vi "lab_3_partie_4.vi"() -> ()   [LabVIEW 2020]
uses:
  <instrlib>/Agilent 34401/Public/Data/Read (Single Point).vi
  <instrlib>/Agilent E363X Series/Agilent E363X Series.lvlib
  <instrlib>/Agilent 34401/Agilent 34401.lvlib
panel:
  out "XY Graph":cluster{"Y":dbl[], "Y":dbl[]}[](graph) caption="Graphe XY"
  in  "Tension maximale":dbl(slide) scale=0.0..6.0
  out "Courant":dbl
  in  "Incrément \ntension":sgl step=0.05
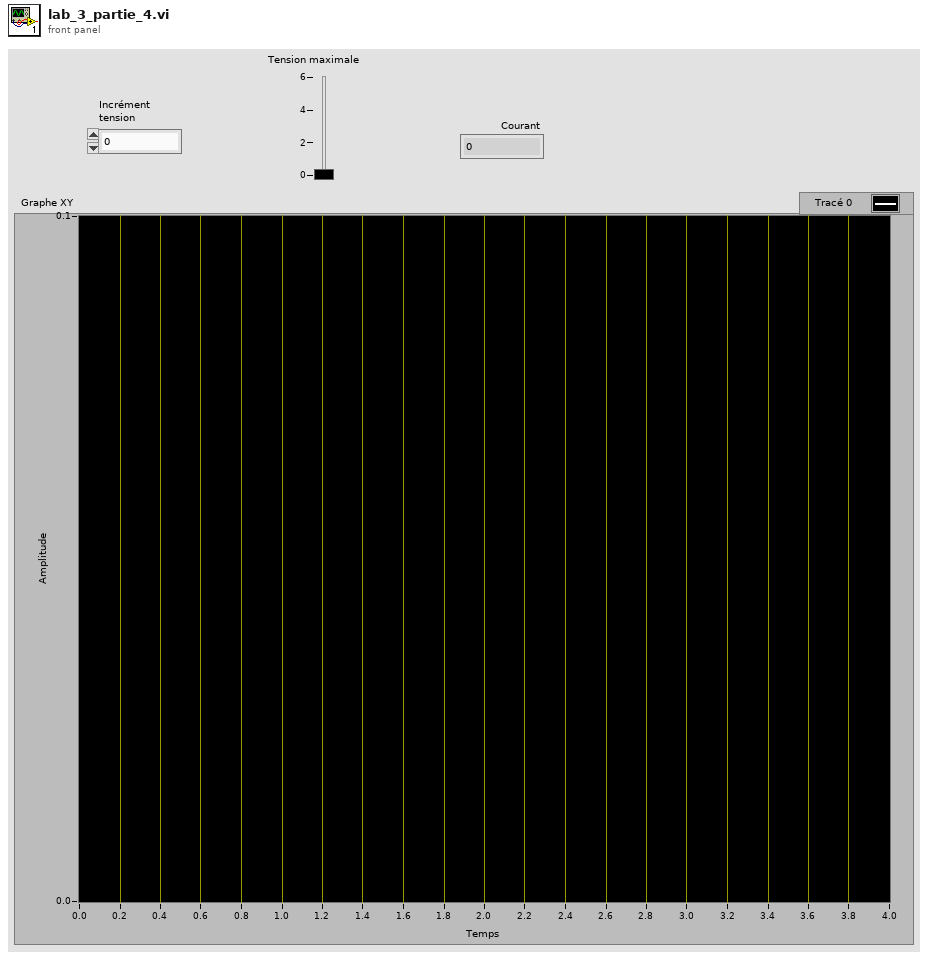
[diagram p1: front panel]
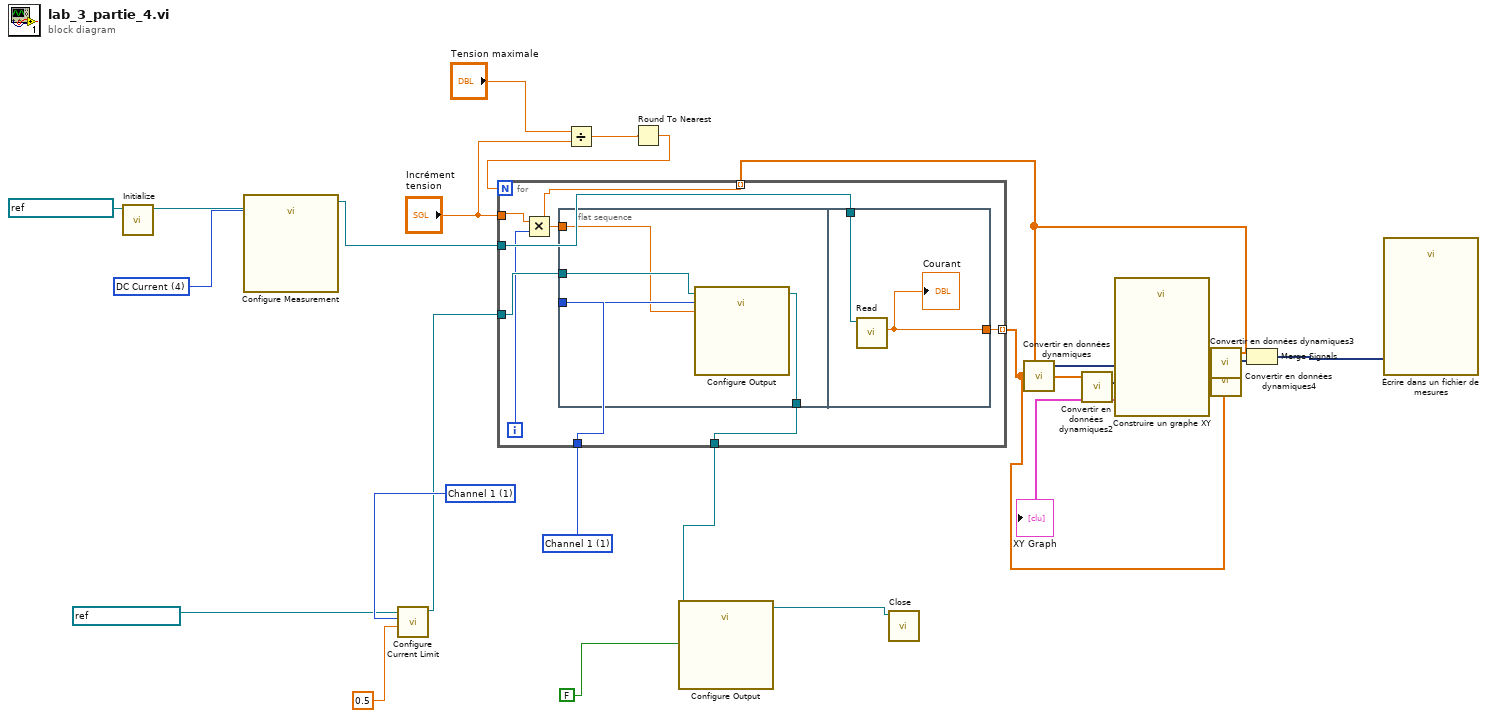
[diagram p0: block diagram]
diagram:
  w20 = u16 4 items=["DC Voltage", "AC Voltage", "2 - Wire Resistance", "4 - Wire Resistance", "DC Current", "AC Current", "Frequency", "Period", "Continuity", "Diode Checking", "VDC:VDC Ratio", "Temperature", "Capacitance"] ("Function (0: DC Voltage)")
  w18 = 1 items=["Channel 1"=1, "Channel 2"=2, "Channel 3"=3] ("Channel (1: Channel 1)")
  w23 = 1 items=["Channel 1"=1, "Channel 2"=2, "Channel 3"=3] ("Channel (1: Channel 1)")
  n1 = call <instrlib>:"Initialize.vi"("VISA resource name"=refnum<visa-resource-name> "GPIB0::22::INSTR") -> ("VISA resource name out"=w21:refnum<visa-resource-name>)  [unwired: 9 in, 1 out]
  n2 = call <instrlib>:"Configure Measurement.vi"("Function (0: DC Voltage)"=w20, "VISA resource name"=w21) -> ("VISA resource name out"=w15:refnum<visa-resource-name>)  [unwired: 8 in, 1 out]
  n3 = call <instrlib>:"Configure Current Limit.vi"("Current Limit (0.0 A)"=0.5, "Channel (1: Channel 1)"=w23, "VISA resource name"=refnum<visa-resource-name> "GPIB0::5::INSTR") -> ("VISA resource name out"=w17:refnum<visa-resource-name>)  [unwired: 7 in, 1 out]
  n4 = Divide(x="Tension maximale", y="Incrément \ntension") -> (x/y=w12:dbl)
  n5 = Round To Nearest(number=w12) -> (nearest integer value=w11:dbl)
  n6 = for {
    N: w11 -> [_]
    tunnel: w18 -> [w32]
    tunnel: w17 -> [w31]
    tunnel: [w30] -> w16
    tunnel: w15 -> [w29]
    tunnel: "Incrément \ntension" -> [w28]
    tunnel: [w26] -> w6 mode=indexing
    tunnel: [w25] -> w4 mode=indexing
    i -> [w27]
    n7 = Multiply(x=w28, y=w27) -> (x*y=w26:sgl)
    n8 = flat-sequence {
      tunnel: w32 -> [w36]
      tunnel: w31 -> [w35]
      tunnel: [w34] -> w30
      tunnel: w26 -> [w33]
      tunnel: w29 -> [w38]
      tunnel: [w37] -> w25
      frame #0 {
        n9 = call <instrlib>:"Configure Output.vi"("Voltage Level (0.0 V)"=w33, "Channel (1: Channel 1)"=w36, "VISA resource name"=w35) -> ("VISA resource name out"=w34:refnum<visa-resource-name>)  [unwired: 7 in, 1 out]
      }
      frame #1 {
        n10 = call-poly <instrlib>:"Read.vi"("VISA resource name"=w38) -> ("Measurement"=w37:dbl)  [unwired: 8 in, 2 out]
        "Courant" <- w37
      }
    }
  }
  n11 = call <instrlib>:"Configure Output.vi"("Enable Output (T: Enable)"=FALSE, "VISA resource name"=w16) -> ("VISA resource name out"=w19:refnum<visa-resource-name>)  [unwired: 8 in, 1 out]
  n12 = call <instrlib>:"Close.vi"("VISA resource name"=w19) -> ()  [unwired: 10 in, 1 out]
  n13 = call "Convertir en données dynamiques"("Array"=w6) -> ("Dynamic Data Type"=w9:dynamicdata)  [unwired: 3 in]
  n14 = call "Convertir en données dynamiques2"("Array"=w4) -> ("Dynamic Data Type"=w8:dynamicdata)  [unwired: 3 in]
  n15 = call "Construire un graphe XY"("Y Input"=w8, "X Input"=w9) -> ("XY Graph"=→"XY Graph":cluster{"X":dbl[], "Y":dbl[]}[])  [unwired: 8 in, 1 out]
  n16 = call "Convertir en données dynamiques3"("Array"=w6) -> ("Dynamic Data Type"=w5:dynamicdata)  [unwired: 3 in]
  n17 = call "Convertir en données dynamiques4"("Array"=w4) -> ("Dynamic Data Type"=w3:dynamicdata)  [unwired: 3 in]
  n18 = Merge Signals(w5, w3) -> (w7:dynamicdata)
  n19 = call "Écrire dans un fichier de mesures"("Signals"=w7) -> ()  [unwired: 16 in, 3 out]
